vi "Sequence Get All.vi"(6 "Descending? (F)":bool, 8 "error in (no error)":errorcluster, 10 "Sort by (sxSequenceId)":T1=enum."sxSequenceId", 11 "Connection Refnum":T2) -> (0 "error out":errorcluster, 1 "Sequence IDs":string[](array[string]), 2 "Sequence Records":T3[](array[typedef]), 3 "Connection Refnum":T2, 4 "Data Present":bool)   [LabVIEW 2011]
uses:
  Sequence Record.ctl
  SI.LIB/ODBC/SQL Controls/Connection Refnum.ctl
  Sequence Fields.ctl
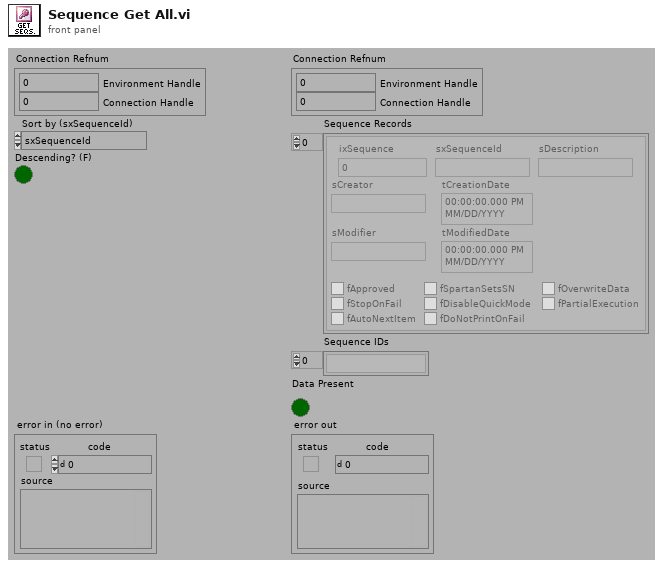
[diagram p1: front panel]
types:
  T1 = typedef "Sequence Fields.ctl" = enum32{"ixSequence", "sxSequenceId", "sDescription", "sCreator", "tCreationDate", "sModifier", "tModifiedDate", "fApproved", "fSpartanSetsSN", "fOverwriteData", "fStopOnFail", "fDisableQuickMode", "fPartialExecution", "fAutoNextItem"}
  T2 = typedef "Connection Refnum.ctl" = cluster{"Environment Handle":i32, "Connection Handle":i32}
  T3 = typedef "Sequence Record.ctl" = cluster{"ixSequence":i32, "sxSequenceId":string, "sDescription":string, "sCreator":string, "tCreationDate":timestamp, "sModifier":string, "tModifiedDate":timestamp, "fApproved":bool, "fSpartanSetsSN":bool, "fOverwriteData":bool, "fStopOnFail":bool, "fDisableQuickMode":bool, "fPartialExecution":bool, "fAutoNextItem":bool, "fDoNotPrintOnFail":bool}
  T4 = typedef "Statement Refnum.ctl" = cluster{"Statement Handle":i32, "Parameter Number":u16}
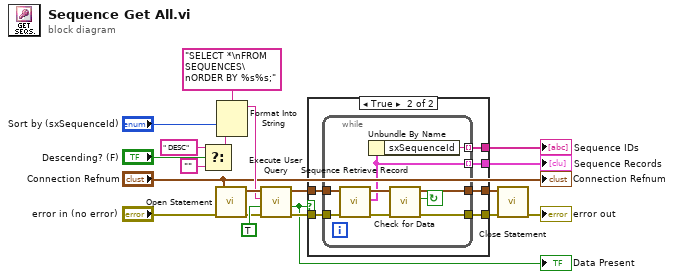
[diagram p0: block diagram]
diagram:
  n1 = Select(t=" DESC" ("input 2"), s="Descending? (F)", f="") -> (s? t:f=w10:string)
  n2 = call "Open Statement.vi"("error in (no error)"="error in (no error)", "Connection Refnum"="Connection Refnum") -> ("error out"=w14:errorcluster, "Statement Refnum"=w15:T4)  [unwired: 4 out]
  n3 = Format Into String(format string="SELECT *\nFROM SEQUENCES\nORDER BY %s%s;" ("Query Name"), "Sort by (sxSequenceId)", w10) -> (resulting string=w6:string)  [unwired: 2 in, 1 out]
  n4 = call "Execute User Query.vi"("error in (no error)"=w14, "Return Data? (f)"=TRUE, "User Query"=w6, "Statement Refnum"=w15) -> ("error out"=w20:errorcluster, "Data Present?"=w13:bool, "Statement Refnum"=w19:T4)  [unwired: 1 out]
  "Data Present" <- w13
  n5 = case shown="True" w13 {
    tunnel: w20 -> [w21 w27]
    tunnel: w19 -> [w22 w28]
    tunnel: [w21 w25] -> w16
    tunnel: [w22 w26] -> w17
    tunnel: [_ w24] -> w3
    tunnel: [_ w23] -> w2
    frame False {
    }
    frame True {
      n6 = while {
        tunnel: w28 -> [w36]
        tunnel: w27 -> [w35]
        tunnel: [w33] -> w26
        tunnel: [w31] -> w25
        tunnel: [w30] -> w23 mode=indexing
        tunnel: [w29] -> w24 mode=indexing
        stop <- w37 continue-if-true
        n7 = call "Sequence Retrieve Record.vi"("error in (no error)"=w35, "Statement Refnum"=w36) -> ("error out"=w32:errorcluster, "Sequence Record"=w30:T3, "Statement Refnum"=w34:T4)  [unwired: 7 out]
        n8 = Unbundle By Name(w30) -> ("sxSequenceId"=w29:string)
        n9 = call "Check for Data.vi"("error in (no error)"=w32, "Statement Refnum"=w34) -> ("error out"=w31:errorcluster, "Data Present?"=w37:bool, "Statement Refnum"=w33:T4)  [unwired: 3 out]
      }
    }
  }
  "Sequence Records" <- w2
  "Sequence IDs" <- w3
  n10 = call "Close Statement.vi"("error in (no error)"=w16, "Statement Refnum"=w17) -> ("error out"=→"error out":errorcluster)  [unwired: 5 out]
  "Connection Refnum" <- "Connection Refnum"
